vi "Lvi Set Timing.vi"(0 "TaskRef":i32, 1 "ClkSource":u32, 2 "SyncMode":u32, 5 "SampleMode":u32, 7 "PointsPerChan":u32, 9 "SampleRate":dbl, 11 "error in (no error)":errorcluster, 12 "NumBuffers":u32) -> (4 "TaskRef out":i32, 6 "ActualSampleRate":dbl, 8 "function return":u32(ring), 15 "error out":errorcluster)   [LabVIEW 2022 SP3, in "DtLvLink.lvlib"]
doc: "Calls directly into the entry points of the DLL of the Data Acq SDK to specify the timing- or clock-related attributes of an analog input or analog output task, and create one or more buffers when needed. This VI is used by the higher-level VI, DtOLTiming."
uses:
  DtLvLink.lvlib
  <userlib>/LV-Link3/DtLvLink_64.dll
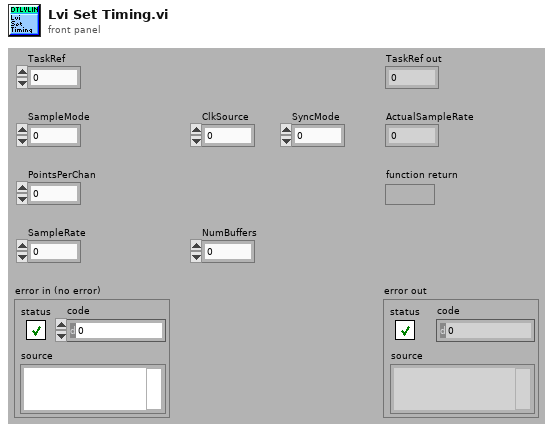
[diagram p1: front panel]
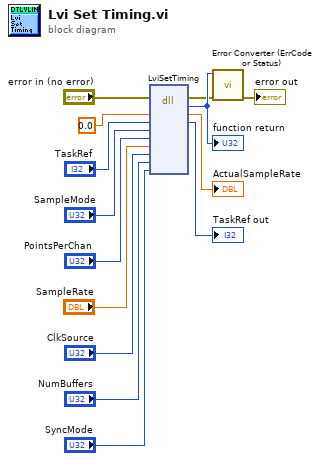
[diagram p0: block diagram]
diagram:
  n1 = dll-call lib="C:/Program Files/National Instruments/LabVIEW 2022/user.lib/LV-Link3/DtLvLink_64.*" fn="LviSetTiming"(error in="error in (no error)", "ActualSampleRate"=0.0, "TaskRef"="TaskRef", "SampleMode"="SampleMode", "PointsPerChan"="PointsPerChan", "SampleRate"="SampleRate", "ClkSource"="ClkSource", "NumBuffers"="NumBuffers", "SyncMode"="SyncMode") -> (error out=w2:errorcluster, w14:u32, "ActualSampleRate"=→"ActualSampleRate":dbl, "TaskRef"=→"TaskRef out":i32)  [unwired: 8 in, 1 out]
  "function return" <- w14
  n2 = call "Error Converter (ErrCode or Status).vi"("error in (no error)"=w2, "error code"=w14) -> ("error out"=→"error out":errorcluster)  [unwired: 9 in]
